vi "视觉浏览器.vi"() -> ()   [LabVIEW 2018]
uses:
  <vilib>/vision/NI_Vision_Development_Module.lvlib
panel:
  out "error out":errorcluster
  out "Image":T1(plugin-control)
  in  "路径":path
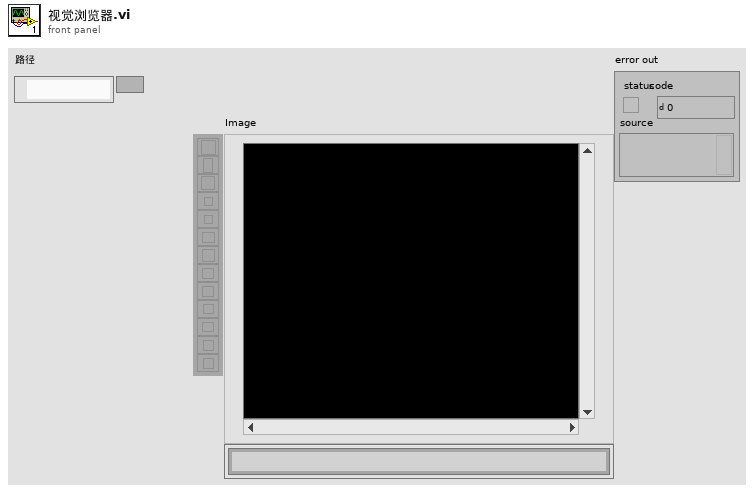
[diagram p1: front panel]
types:
  T1 = typedef "IMAQ Image.ctl" = refnum<image>
  T2 = typedef "Image Type" = u32
  T3 = cluster{"Browser Size":cluster{"X":i32, "Y":i32}, "Images per Line":i32, "Background Color":u32, "Frame Size":i32, "Frame Style":enum16{"Raised", "Bevelled", "Outline", "Hidden", "Step", "Raised Outline"}}
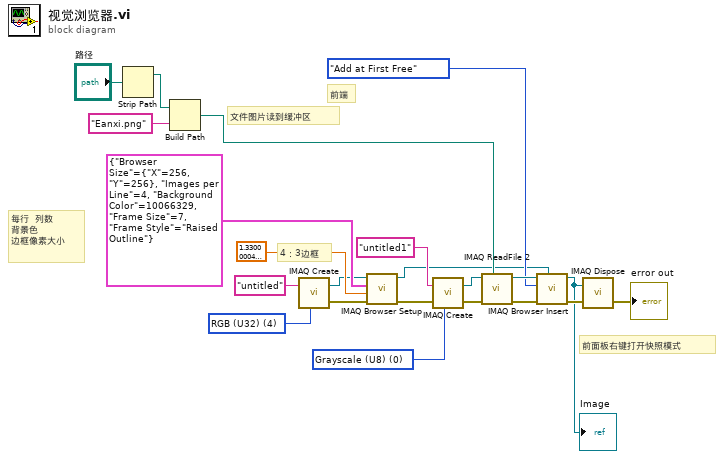
[diagram p0: block diagram]
diagram:
  w9 = T2 0 items=["Grayscale (U8)", "Grayscale (I16)", "Grayscale (SGL)", "Complex (CSG)", "RGB (U32)", "HSL (U32)", "RGB (U64)", "Grayscale (U16)"] ("Image Type")
  w20 = T2 4 items=["Grayscale (U8)", "Grayscale (I16)", "Grayscale (SGL)", "Complex (CSG)", "RGB (U32)", "HSL (U32)", "RGB (U64)", "Grayscale (U16)"] ("Image Type")
  # "每行  列数\n背景色\n边框像素大小"
  # "前面板右键打开快照模式"
  # "前端"
  # "文件图片读到缓冲区"
  # "4：3边框"
  n1 = Strip Path(path="路径") -> (stripped path=w15:path)  [unwired: 1 out]
  n2 = Build Path(base path=w15, name or relative path="Eanxi.png" ("名称或相对路径")) -> (appended path=w8:path)
  n3 = call "IMAQ Create"("Image Name"="untitled", "Image Type"=w20) -> ("New Image"=w18:T1, "error out"=w17:errorcluster)  [unwired: 3 in]
  n4 = call "IMAQ Browser Setup"("error in (no error)"=w17, "Image Ratio"=sgl 1.33, "Browser Info"=T3 {"Browser Size"={"X"=256, "Y"=256}, "Images per Line"=4, "Background Color"=10066329, "Frame Size"=7, "Frame Style"=enum."Raised Outline"}, "Image In"=w18) -> ("error out"=w10:errorcluster, "Image Browser Out"=w4:T1)  [unwired: 2 out]
  n5 = call "IMAQ Create"("Image Name"="untitled1", "Image Type"=w9, "error in (no error)"=w10) -> ("New Image"=w13:T1, "error out"=w11:errorcluster)  [unwired: 2 in]
  n6 = call "IMAQ ReadFile 2"("File Path"=w8, "error in (no error)"=w11, "Image"=w13) -> ("error out"=w6:errorcluster, "Image Out"=w7:T1)  [unwired: 4 in, 3 out]
  n7 = call "IMAQ Browser Insert"("Image Browser In"=w4, "error in (no error)"=w6, "Insertion Mode"=enum16{"Add at First Free", "Add at the End"}."Add at First Free", "Image to Add"=w7) -> ("error out"=w3:errorcluster, "Image Browser Out"=w2:T1)  [unwired: 3 in, 3 out]
  "Image" <- w2
  n8 = call "IMAQ Dispose"("Image"=w2, "error in (no error)"=w3) -> ("error out"=→"error out":errorcluster)  [unwired: 4 in]
